vi "Define.vi"(11 "Relation Definition":T1) -> (3 "Entity Collection out":refnum<class "Entity Collection.lvclass">)   [LabVIEW 2022 SP3, in "Conditum.lvlib" / "Columns.lvlib" / "Entity Collection.lvclass"]
uses:
  Entity Collection.lvclass
  Entity Collection.lvclass/Entity Collection.ctl
  Relation/Relation.lvclass
  C:/dev/lv/illuminated-g/lv-conditum/Conditum/Columns/Relation/Relation.lvclass
  C:/dev/lv/illuminated-g/lv-conditum/Conditum/Columns/Type/Type.lvclass
  C:/dev/lv/illuminated-g/lv-conditum/Conditum/Columns/Entity Collection/Entity Collection.lvclass
  Type/Definition.ctl
  Type/Type.lvclass
  Entity/Entity.lvclass
  Relation Mapping.ctl
  Conditum.lvlib
  Relation/Definition.ctl
  Relation/Relation Definition.ctl
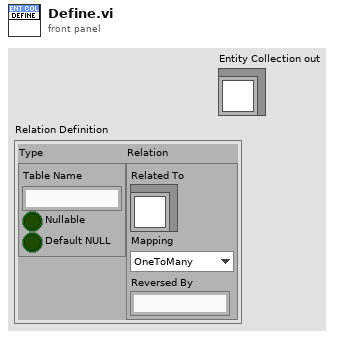
[diagram p1: front panel]
types:
  T1 = typedef "Conditum.lvlib/Columns.lvlib/Relation.lvclass/Relation Definition.ctl" = cluster{"Type":T2, "Relation":T3}
  T2 = typedef "Conditum.lvlib/Columns.lvlib/Type.lvclass/Definition.ctl" = cluster{"Table Name":string, "Nullable":bool, "Default NULL":bool}
  T3 = typedef "Conditum.lvlib/Columns.lvlib/Relation.lvclass/Definition.ctl" = cluster{"Related To":refnum<class "Entity.lvclass">, "Mapping":T4, "Reversed By":string}
  T4 = typedef "Conditum.lvlib/Relation Mapping.ctl" = enum16{"OneToMany", "ManyToOne", "ManyToMany", "OneToOne"}
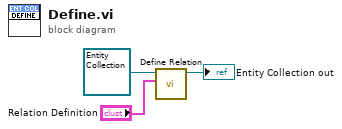
[diagram p0: block diagram]
diagram:
  n1 = call "Define Relation.vi"("Relation Definition"="Relation Definition", "Relation in"=refnum<class "Entity Collection.lvclass"> refnum ("Entity Collection in")) -> ("Relation out"=→"Entity Collection out":refnum<class "Entity Collection.lvclass">)  [unwired: 9 in]
